vi "Determine Periodic.vi"(6 "Generation Counter":u32, 8 "Generation Iterations":u32, 9 "Generation Period":u32, 10 "Time Since Last Generation in":u32, 11 "Current Time":u32) -> (1 "Tranmit":bool, 2 "Generation Counter out":u32, 3 "Time Since Last Generation out":u32)   [LabVIEW 2024, in "Protection and Counter Support Engine.lvlib"]
uses:
  Protection and Counter Support Engine.lvlib
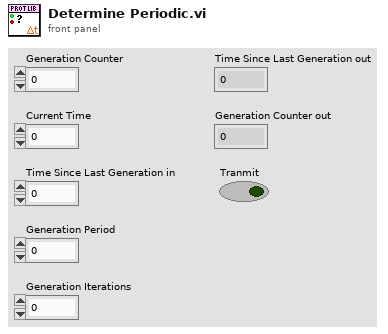
[diagram p1: front panel]
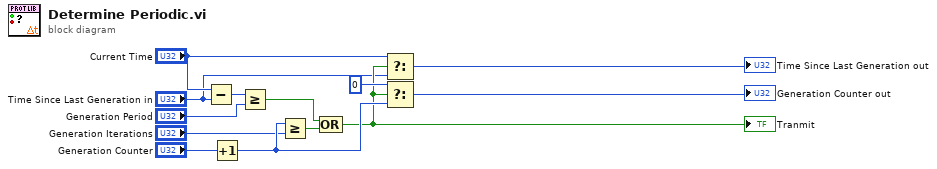
[diagram p0: block diagram]
diagram:
  n1 = Subtract(x="Current Time", y="Time Since Last Generation in") -> (x-y=w9:u32)
  n2 = Increment(x="Generation Counter") -> (x+1=w12:u32)
  n3 = Greater Or Equal?(x=w9, y="Generation Period") -> (x >= y?=w11:bool)
  n4 = Greater Or Equal?(x=w12, y="Generation Iterations") -> (x >= y?=w10:bool)
  n5 = Compound Arithmetic op=OR(w11, w10) -> (w7:bool)
  "Tranmit" <- w7
  n6 = Select(t="Current Time", s=w7, f="Time Since Last Generation in") -> (s? t:f=→"Time Since Last Generation out":u32)
  n7 = Select(t=u32 0, s=w7, f=w12) -> (s? t:f=→"Generation Counter out":u32)
